vi "Set File Properties.vi"(8 "error in (no error)":errorcluster, 11 "Data Logger Module in":refnum<class "Data Logger Module.lvclass">) -> (0 "error out":errorcluster, 3 "Data Logger Module out":refnum<class "Data Logger Module.lvclass">)   [LabVIEW 2020, in "VolatusData.lvlib" / "Data Logger Module.lvclass"]
uses:
  Data Logger Module.lvclass
  C:/dev/lv20CE/relink/lv-volatus/Volatus/Module/Module.lvclass
  Data Logger Module.lvclass/Data Logger Module.ctl
  Volatus/Module/Module.lvclass
  C:/dev/lv20CE/relink/lv-volatus/VolatusData/Data Logger Module/Data Logger Module.lvclass
  Volatus/VolatusAPI/VolatusAPI.lvclass
  VolatusConfig/VolatusConfig/VolatusConfig.lvclass
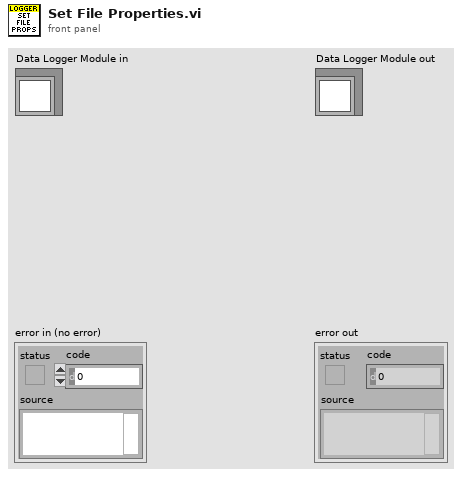
[diagram p1: front panel]
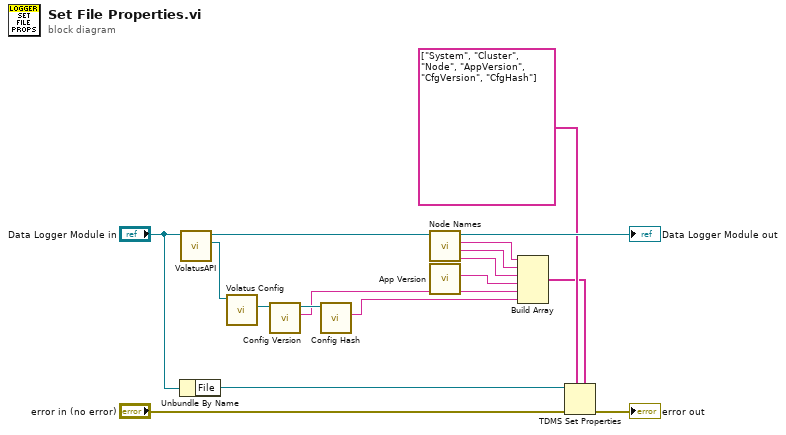
[diagram p0: block diagram]
diagram:
  n1 = Unbundle By Name("Data Logger Module in") -> ("File"=w15:refnum<k34>)
  n2 = call "VolatusAPI.vi"("Module in"="Data Logger Module in") -> ("VolatusAPI"=w5:refnum<class "VolatusAPI.lvclass">, "Module out"=w7:refnum<class "Data Logger Module.lvclass">)  [unwired: 9 in]
  n3 = call "Volatus Config.vi"("VolatusAPI in"=w5) -> ("Volatus Config"=w4:refnum<class "VolatusConfig.lvclass">)  [unwired: 8 in, 2 out]
  n4 = call "Config Version.vi"("VolatusConfig in"=w4) -> ("Config Version"=w2:string, "VolatusConfig out"=w3:refnum<class "VolatusConfig.lvclass">)  [unwired: 8 in, 1 out]
  n5 = call "Config Hash.vi"("VolatusConfig in"=w3) -> ("Config Hash"=w1:string)  [unwired: 8 in, 2 out]
  n6 = call "Node Names.vi"("Module in"=w7) -> ("Node"=w9:string, "Cluster"=w10:string, "System"=w11:string, "Module out"=→"Data Logger Module out":refnum<class "Data Logger Module.lvclass">)  [unwired: 6 in, 1 out]
  n7 = call "App Version.vi"() -> ("App Version"=w6:string)  [unwired: 11 in]
  n8 = Build Array(w11, w10, w9, w6, w2, w1) -> (w8:string[])
  n9 = TDMS Set Properties(5:w8, 7:string[] ["System", "Cluster", "Node", "AppVersion", "CfgVersion", "CfgHash"], 8:"error in (no error)", 11:w15) -> (0:→"error out":errorcluster)  [unwired: 2 in, 3 out]
